vi "test Increment.vi"(8 "error in (no error)":errorcluster, 11 "TestCase in":refnum<class "Configuration Tests.lvclass">) -> (0 "error out":errorcluster, 3 "TestCase out":refnum<class "Configuration Tests.lvclass">)   [LabVIEW 2017, in "Configuration Tests.lvclass"]
uses:
  Configuration Tests.lvclass
  Engine/Classes/Transfer Group/Transfer Group.lvclass
  Engine/Classes/Plugin/Plugin.lvclass
  Engine/Classes/Plugin/Plugin.lvclass/Plugin.ctl
  Engine/Classes/Timing/Timing.lvclass/Timing.ctl
  Engine/Classes/Transfer Group/Transfer Group.lvclass/Transfer Group.ctl
  <vilib>/addons/_JKI Toolkits/VI Tester/TestCase.llb/TestCase.lvclass
  Engine/Classes/Timing/Timing.lvclass
  C:/Program Files (x86)/National Instruments/LabVIEW 2017/vi.lib/addons/_JKI Toolkits/VI Tester/TestCase.llb/TestCase.lvclass
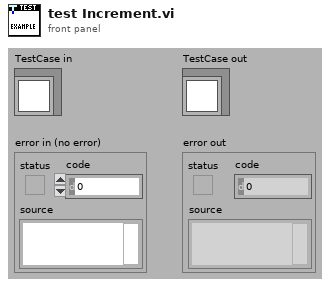
[diagram p1: front panel]
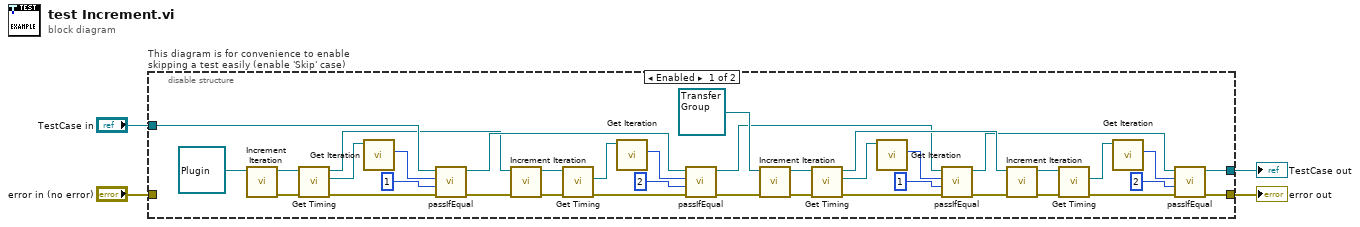
[diagram p0: block diagram]
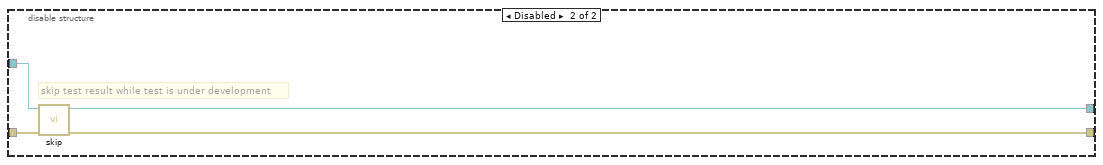
[diagram p2: hidden frame]
diagram:
  n1 = disable-structure "This diagram is for convenience to enable skipping a test easily (enable 'Skip' case)" shown="Enabled" {
    disable-tunnel: "TestCase in" -> [w34 w41]
    disable-tunnel: [w5 w39] -> w1
    disable-tunnel: [w7 w40] -> w3
    disable-tunnel: "error in (no error)" -> [_ w38]
    frame Enabled {
      n2 = call "Increment Iteration.vi"("Plugin in"=refnum<class "Plugin.lvclass"> refnum) -> ("error out"=w35:errorcluster, "Plugin out"=w37:refnum<class "Plugin.lvclass">)  [unwired: 9 in]
      n3 = call "Get Timing.vi"("Plugin in"=w37) -> ("Timing"=w36:refnum<class "Timing.lvclass">, "Plugin out"=w24:refnum<class "Plugin.lvclass">)  [unwired: 9 in]
      n4 = call "Get Iteration.vi"("Timing in"=w36) -> ("Iteration"=w33:u64)  [unwired: 9 in, 1 out]
      n5 = call-dynamic "passIfEqual.vi"("error in (no error)"=w35, "y"=u64 1 ("Iteration"), "x"=w33, "TestCase in"=w34) -> ("error out"=w26:errorcluster, "TestCase out"=w27:refnum<class "Configuration Tests.lvclass">)  [unwired: 6 in]
      n6 = call "Increment Iteration.vi"("error in (no error)"=w26, "Plugin in"=w24) -> ("error out"=w25:errorcluster, "Plugin out"=w28:refnum<class "Plugin.lvclass">)  [unwired: 8 in]
      n7 = call "Get Timing.vi"("Plugin in"=w28) -> ("Timing"=w29:refnum<class "Timing.lvclass">)  [unwired: 9 in, 1 out]
      n8 = call "Get Iteration.vi"("Timing in"=w29) -> ("Iteration"=w30:u64)  [unwired: 9 in, 1 out]
      n9 = call-dynamic "passIfEqual.vi"("error in (no error)"=w25, "y"=u64 2 ("Iteration"), "x"=w30, "TestCase in"=w27) -> ("error out"=w8:errorcluster, "TestCase out"=w6:refnum<class "Configuration Tests.lvclass">)  [unwired: 6 in]
      n10 = call "Increment Iteration.vi"("error in (no error)"=w8, "Transfer Group in"=refnum<class "Transfer Group.lvclass"> refnum ("DSF.Engine.lvlib:DSF.Engine.Transfer Group.lvclass")) -> ("error out"=w12:errorcluster, "Transfer Group out"=w10:refnum<class "Transfer Group.lvclass">)  [unwired: 8 in]
      n11 = call "Get Timing.vi"("Transfer Group in"=w10) -> ("Timing"=w11:refnum<class "Timing.lvclass">, "Transfer Group out"=w22:refnum<class "Transfer Group.lvclass">)  [unwired: 9 in]
      n12 = call "Get Iteration.vi"("Timing in"=w11) -> ("Iteration"=w13:u64)  [unwired: 9 in, 1 out]
      n13 = call-dynamic "passIfEqual.vi"("error in (no error)"=w12, "y"=u64 1 ("Iteration"), "x"=w13, "TestCase in"=w6) -> ("error out"=w20:errorcluster, "TestCase out"=w19:refnum<class "Configuration Tests.lvclass">)  [unwired: 6 in]
      n14 = call "Increment Iteration.vi"("error in (no error)"=w20, "Transfer Group in"=w22) -> ("error out"=w21:errorcluster, "Transfer Group out"=w18:refnum<class "Transfer Group.lvclass">)  [unwired: 8 in]
      n15 = call "Get Timing.vi"("Transfer Group in"=w18) -> ("Timing"=w17:refnum<class "Timing.lvclass">)  [unwired: 9 in, 1 out]
      n16 = call "Get Iteration.vi"("Timing in"=w17) -> ("Iteration"=w16:u64)  [unwired: 9 in, 1 out]
      n17 = call-dynamic "passIfEqual.vi"("error in (no error)"=w21, "y"=u64 2 ("Iteration"), "x"=w16, "TestCase in"=w19) -> ("error out"=w7:errorcluster, "TestCase out"=w5:refnum<class "Configuration Tests.lvclass">)  [unwired: 6 in]
    }
    frame Disabled {
      # "skip test result while test is under development"
      n18 = call <vilib>:"skip.vi"("error in (no error)"=w38, "TestCase in"=w41) -> ("error out"=w40:errorcluster, "TestCase out"=w39:refnum<class "Configuration Tests.lvclass">)  [unwired: 8 in]
    }
  }
  "error out" <- w3
  "TestCase out" <- w1
